vi "Write Time Stamp.vi"(8 "error in (no error)":errorcluster, 10 "Time Stamp":timestamp, 11 "Timestamp Result in":refnum<class "Timestamp Result.lvclass">) -> (0 "error out":errorcluster, 3 "Timestamp Result out":refnum<class "Timestamp Result.lvclass">)   [LabVIEW 2015, in "Timestamp Result.lvclass"]
uses:
  Timestamp Result.lvclass
  Timestamp Result.lvclass/Timestamp Result.ctl
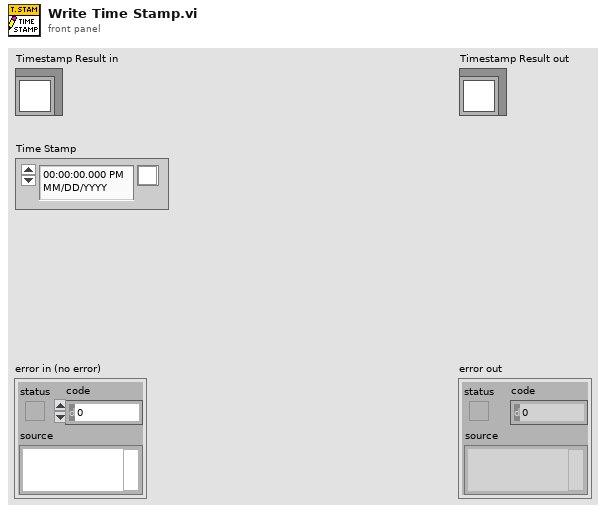
[diagram p1: front panel]
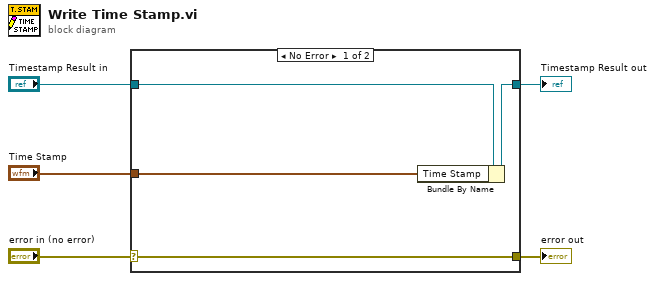
[diagram p0: block diagram]
diagram:
  n1 = case shown="No Error" "error in (no error)" {
    selector: "error in (no error)" -> [w9 w10]
    tunnel: [w9 w10] -> w4
    tunnel: [w7 w11] -> w2
    tunnel: "Timestamp Result in" -> [w8 w11]
    tunnel: "Time Stamp" -> [w6 _]
    frame No Error {
      n2 = Bundle By Name(cluster=w8, "Time Stamp"=w6) -> (w7:refnum<class "Timestamp Result.lvclass">)
    }
    frame Error {
    }
  }
  "error out" <- w4
  "Timestamp Result out" <- w2
